vi "SetPowerRange.vi"(2 "Power to Measure (0.0)":dbl, 3 "resource name":string="USB0::0x1313::0x8078::P0005368::INSTR") -> (0 "error out":errorcluster {"code" format="%.0x"})   [LabVIEW 2015]
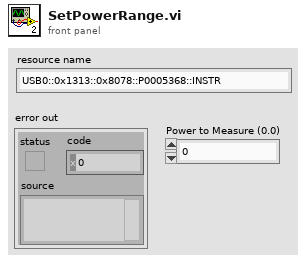
[diagram p1: front panel]
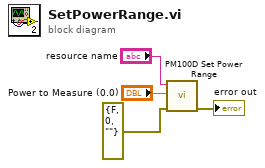
[diagram p0: block diagram]
diagram:
  n1 = call "PM100D Set Power Range.vi"("error in (no error)"=errorcluster {"status"=FALSE, "code"=0, "source"=""}, "Power to Measure (0.0)"="Power to Measure (0.0)", "instrument handle"="resource name") -> ("error out"=→"error out":errorcluster)  [unwired: 7 in, 1 out]
